vi "Configure Std Waveform.vi"(8 "error in":errorcluster, 11 "FGen PXI Base CFG in":refnum<class "Generate DC CFG.lvclass">) -> (0 "error out":errorcluster, 3 "FGen PXI Base CFG out":refnum<class "Generate DC CFG.lvclass">)   [LabVIEW 2023, in "FGen Simulated CFGs.lvlib" / "Generate DC CFG.lvclass"]
uses:
  Generate DC CFG.lvclass
  Configuration/Configuration JSON/Configuration JSON Base/CFG JSON.lvclass/CFG JSON.ctl
  de57daef-5d54-4cfc-861f-41c83b56b32c.vi
  <vilib>/JDP Science/JSONtext/Find Item.vi
  <vilib>/JDP Science/JSONtext/Next JSON Value.vi
  <vilib>/JDP Science/JSONtext/String Subset.vi
  <vilib>/JDP Science/JSONtext/Parsing/Advance past next JSON Value (inlined COPY).vi
  <vilib>/JDP Science/JSONtext/Parsing/Advance past whitespace.vi
  <vilib>/JDP Science/JSONtext/Parsing/Advance past String.vi
  <vilib>/JDP Science/JSONtext/Parsing/Advance past Number.vi
  <vilib>/JDP Science/JSONtext/Parsing/Advance past Line Ending.vi
  <vilib>/JDP Science/JSONtext/Parsing/Parse Full Path or Item Name.vi
  <vilib>/JDP Science/JSONtext/Parsing/Advance past Array.vi
  <vilib>/JDP Science/JSONtext/Parsing/Advance past Object.vi
  <vilib>/JDP Science/JSONtext/support/Error Cluster From Code.vi
  <vilib>/JDP Science/JSONtext/Offset/Find Item Locations by Path.vi
  <vilib>/JDP Science/JSONtext/JSON text to Variant.vi
  <vilib>/Utility/error.llb/Error Cluster From Error Code.vi
  <vilib>/JDP Science/JSONtext/LVClass Serializer/JSONtext LVClass Serializer.lvclass
  <vilib>/ErrorRing/Error Ring.xnode
  Generate DC CFG.lvclass/Generate DC CFG.ctl
  Configuration/Configuration JSON/Configuration JSON Base/CFG JSON.lvclass
panel:
  out "Data":T1(array[cluster])
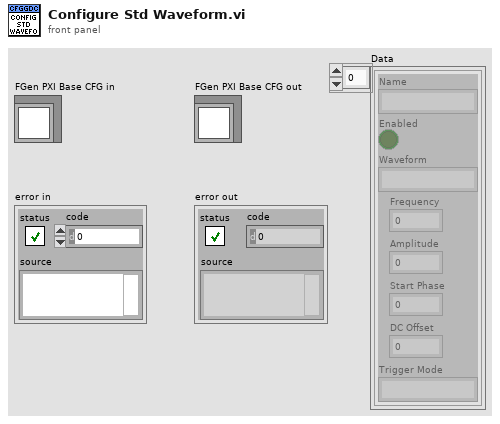
[diagram p1: front panel]
types:
  T1 = cluster{"Name":string, "Enabled":bool, "Waveform":string, "Frequency":dbl, "Amplitude":dbl, "Start Phase":dbl, "DC Offset":dbl, "Trigger Mode":string}[]
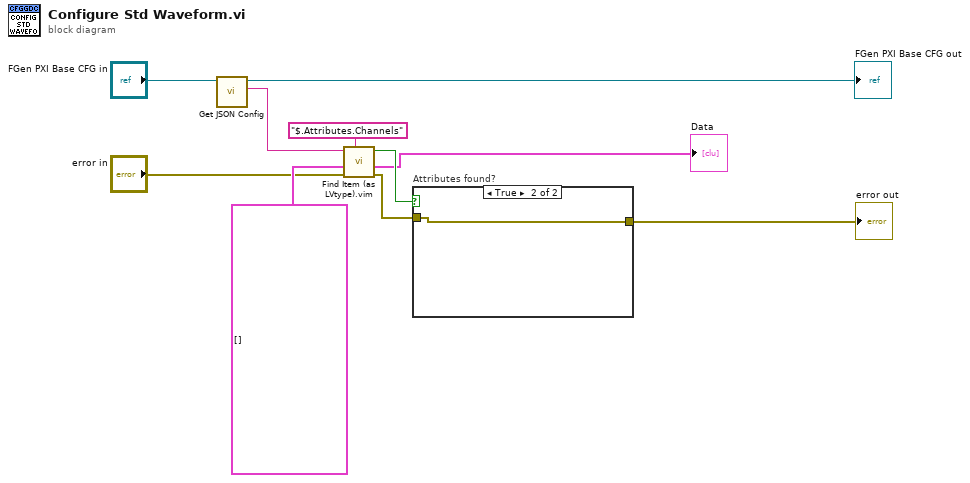
[diagram p0: block diagram]
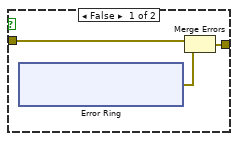
[diagram p2: hidden frame]
diagram:
  n1 = call "Get JSON Config.vi"("CFG Base in"="FGen PXI Base CFG in") -> ("<JSON>Config>"=w5:string, "CFG Base out"=→"FGen PXI Base CFG out":refnum<class "Generate DC CFG.lvclass">)  [unwired: 9 in]
  n2 = call "Find Item (as LVtype).vim"("$Path or Item Name"="$.Attributes.Channels", "error in (no error)"="error in", "Data Type and Default Value"=T1 [], "JSON"=w5) -> ("error out"=w3:errorcluster, "Data"=→"Data":T1, "Found"=w4:bool)  [unwired: 4 in, 1 out]
  n3 = case "Attributes found?" shown="True" w4 {
    tunnel: w3 -> [w12 w19]
    tunnel: [w11 w19] -> w8
    frame False {
      n4 = xnode "Error Ring"() -> ("error out"=w13:errorcluster)
      n5 = Merge Errors(w12, w13) -> (w11:errorcluster)
    }
    frame True {
    }
  }
  "error out" <- w8
